vi "Test golpi Package Installation.vi"() -> ()   [LabVIEW 2020, in "GOLPI library.lvlib"]
doc: "Only for testing of package installation.\n\n---\nGOLPI works only with lv_proc.dll library, which is part of vipm package or should be delivered together with packed library. Placement of this dll is selected in terminal of Start GNU Octave.vi."
uses:
  GOLPI library.lvlib
  Get Struct.vi
  Get Double.vi
panel:
  out "value":dbl format="%.2f"
  in  "quit":bool
  in  "what to test":enum16{"bitstream", "get struct"}(ring)
  in  "Cluster":cluster{"b":dbl, "c":string}
  out "read buffer 1":string
  in  "octave exe file or directory":path
  out "GNU Octave version":string
  out "exit code":i32
  out "error out":errorcluster
  out "pkg list after":string
  in  "working directory":path=path "C:/Users/labina/Documents"
  # "What it does:\n\nUninstall package\nSets bitstream/struct transfer\nChecks installed packages"
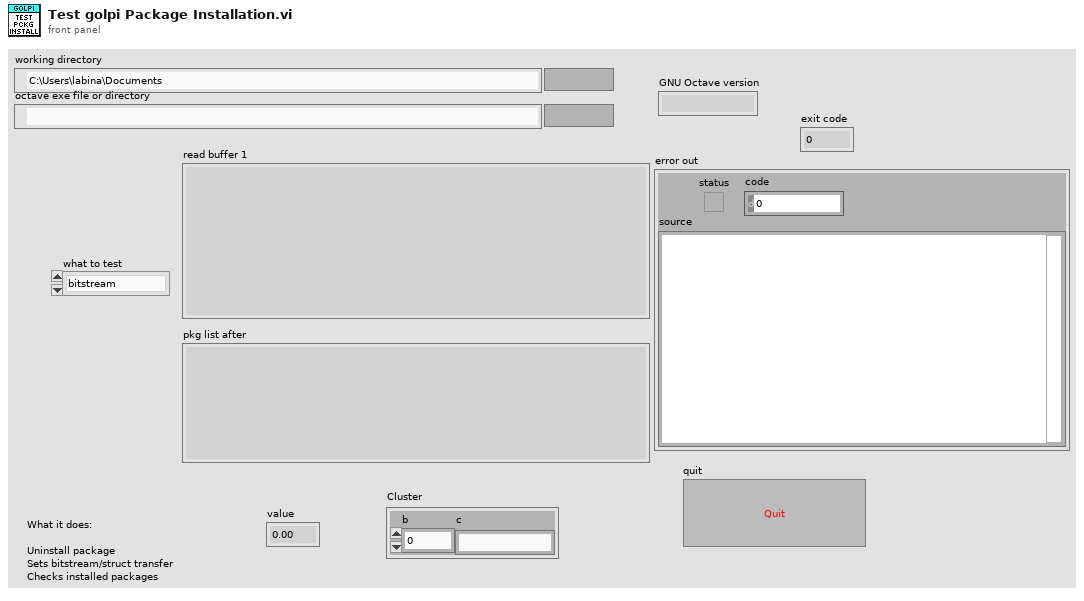
[diagram p1: front panel]
types:
  T1 = typedef "GOLPI library.lvlib/GOLPI reference Type Def.ctl" = cluster{"pipe handle":T2, "fast read timeout [ms]":u32, "fast read settle time [ms]":u32, "fast read to multiple [ms]":u32, "max elements per input line":u32, "slow read timeout [ms]":u32, "stdin double format specifier":string, "max elements per stdout output column":u32, "console mode bitstream":bool, "bitstream first read timeout [ms]":u32, "bitstream read timeout [ms]":u32, "struct transfer possible":bool, "matlab mode":bool}
  T2 = typedef "LV Process library.lvlib/Pipe Handle.ctl" = cluster{"lv_proc.dll file path":path, "process instance handle":u32[], "debug mode":bool, "debug data":cluster{"time":timestamp, "stdin":bool, "data":string}[]}
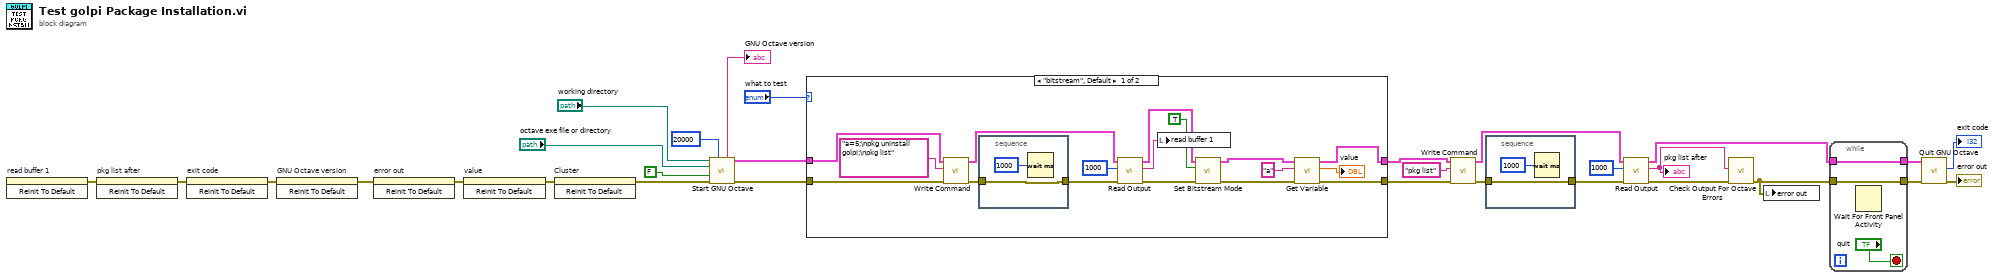
[diagram p0: block diagram]
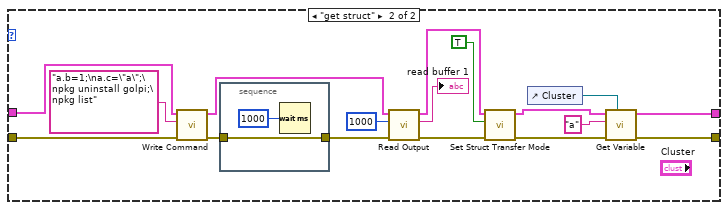
[diagram p2: hidden frame]
diagram:
  n1 = invoke on="read buffer 1" class="Str" method="Reinit To Default"() -> (error out=w5:errorcluster)  [unwired: 3 in, 2 out]
  n2 = invoke on="pkg list after" class="Str" method="Reinit To Default"(error in=w5) -> (error out=w4:errorcluster)  [unwired: 2 in, 2 out]
  n3 = invoke on="exit code" class="DigNum (strict)" method="Reinit To Default"(error in=w4) -> (error out=w7:errorcluster)  [unwired: 2 in, 2 out]
  n4 = invoke on="GNU Octave version" class="Str" method="Reinit To Default"(error in=w7) -> (error out=w8:errorcluster)  [unwired: 2 in, 2 out]
  n5 = invoke on="error out" class="Clust (strict)" method="Reinit To Default"(error in=w8) -> (error out=w9:errorcluster)  [unwired: 2 in, 2 out]
  n6 = invoke on="value" class="DigNum (strict)" method="Reinit To Default"(error in=w9) -> (error out=w10:errorcluster)  [unwired: 2 in, 2 out]
  n7 = invoke on="Cluster" class="Clust (strict)" method="Reinit To Default"(error in=w10) -> (error out=w6:errorcluster)  [unwired: 2 in, 2 out]
  n8 = call "Start GNU Octave.vi"("working dir (user home)"="working directory", "full start timeout [ms] (20000)"=u32 20000 ("Full start timeout [ms] (5000)"), "octave binary file or dir (autofind)"="octave exe file or directory", "hide debug console (T)"=FALSE, "error in"=w6) -> ("GNU Octave version"=→"GNU Octave version":string, "GOLPI ref. out"=w16:T1, "error out"=w17:errorcluster)  [unwired: 7 in, 1 out]
  n9 = case shown="\"bitstream\", Default" "what to test" {
    tunnel: w17 -> [w39 w64]
    tunnel: w16 -> [w40 w62]
    tunnel: [w34 w58] -> w14
    tunnel: [w33 w55] -> w13
    frame "bitstream", Default {
      n10 = call "Write Command.vi"("error in"=w39, "command"="a=5;\npkg uninstall golpi;\npkg list" ("command 1"), "GOLPI ref. in"=w40) -> ("error out"=w44:errorcluster, "GOLPI ref. out"=w43:T1)  [unwired: 7 in]
      n11 = stacked-sequence {
        tunnel: [w48] -> w45
        tunnel: w44 -> [w48]
        frame #0 {
          n12 = Wait (ms)(milliseconds to wait=u32 1000) -> ()  [unwired: 1 out]
        }
      }
      n13 = call "Read Output.vi"("error in"=w45, "byte count"=1000, "GOLPI ref. in"=w43) -> ("error out"=w47:errorcluster, "read buffer"=w38:string, "GOLPI ref. out"=w46:T1)  [unwired: 5 in, 1 out]
      n14 = local write "read buffer 1"(w38) -> ()
      n15 = call "Set Bitstream Mode.vi"("error in"=w47, "Bitstream mode (F)"=TRUE, "GOLPI ref. in"=w46) -> ("error out"=w36:errorcluster, "GOLPI ref. out"=w35:T1)  [unwired: 7 in]
      n16 = call-poly "Get Variable.vi"("error in"=w36, "variable name"="a", "GOLPI ref. in"=w35) -> ("error out"=w33:errorcluster, "value"=→"value":dbl, "GOLPI ref. out"=w34:T1)  [unwired: 6 in]
    }
    frame "get struct" {
      n17 = call "Write Command.vi"("error in"=w64, "command"="a.b=1;\na.c=\"a\";\npkg uninstall golpi;\npkg list" ("command 1"), "GOLPI ref. in"=w62) -> ("error out"=w65:errorcluster, "GOLPI ref. out"=w63:T1)  [unwired: 7 in]
      n18 = stacked-sequence {
        tunnel: [w67] -> w66
        tunnel: w65 -> [w67]
        frame #0 {
          n19 = Wait (ms)(milliseconds to wait=u32 1000) -> ()  [unwired: 1 out]
        }
      }
      n20 = call "Read Output.vi"("error in"=w66, "byte count"=1000, "GOLPI ref. in"=w63) -> ("error out"=w52:errorcluster, "read buffer"=→"read buffer 1":string, "GOLPI ref. out"=w54:T1)  [unwired: 5 in, 1 out]
      n21 = call "Set Struct Transfer Mode.vi"("error in"=w52, "Allow struct tranfer (False)"=TRUE, "GOLPI ref. in"=w54) -> ("error out"=w51:errorcluster, "GOLPI ref. out"=w53:T1)  [unwired: 6 in, 1 out]
      n22 = control-ref of="Cluster"() -> (w56:refnum<vi>)
      n23 = call-poly "Get Variable.vi"("cluster ref (empty)"=w56, "error in"=w51, "variable"="a", "GOLPI ref in"=w53) -> ("error out"=w55:errorcluster, "GOLPI ref. out"=w58:T1)  [unwired: 5 in, 1 out]
    }
  }
  n24 = call "Write Command.vi"("error in"=w13, "command"="pkg list", "GOLPI ref. in"=w14) -> ("error out"=w28:errorcluster, "GOLPI ref. out"=w29:T1)  [unwired: 7 in]
  n25 = stacked-sequence {
    tunnel: [w69] -> w27
    tunnel: w28 -> [w69]
    frame #0 {
      n26 = Wait (ms)(milliseconds to wait=u32 1000) -> ()  [unwired: 1 out]
    }
  }
  n27 = call "Read Output.vi"("error in"=w27, "byte count"=1000, "GOLPI ref. in"=w29) -> ("error out"=w20:errorcluster, "read buffer"=w21:string, "GOLPI ref. out"=w2:T1)  [unwired: 5 in, 1 out]
  "pkg list after" <- w21
  n28 = call "Check Output For Octave Errors.vi"("error in"=w20, "read buffer"=w21) -> ("error out"=w11:errorcluster)  [unwired: 9 in]
  n29 = local write "error out"(w11) -> ()
  n30 = while {
    tunnel: w11 -> [w71]
    tunnel: [w72] -> w3
    tunnel: w2 -> [w72]
    tunnel: [w71] -> w1
    stop <- "quit" stop-if-true
    n31 = Wait For Front Panel Activity() -> ()  [unwired: 3 in, 1 out]
  }
  n32 = call "Quit GNU Octave.vi"("error in"=w1, "GOLPI ref. in"=w3) -> ("error out"=→"error out":errorcluster, "exit code"=→"exit code":i32)  [unwired: 8 in]
